vi "getAllRefs.vi"(8 "error in (no error)":errorcluster, 10 "Language":u8, 11 "Change Language":bool) -> (0 "error out":errorcluster, 3 "Control references [ ]":T1(array[cluster]))   [LabVIEW 2013, in "main.lvlib"]
uses:
  main.lvlib
  <userlib>/_OpenG.lib/file/file.llb/File Exists - Scalar__ogtk.vi
  <vilib>/Utility/file.llb/Read From Spreadsheet File (string).vi
  <vilib>/Utility/file.llb/Write To Spreadsheet File (string).vi
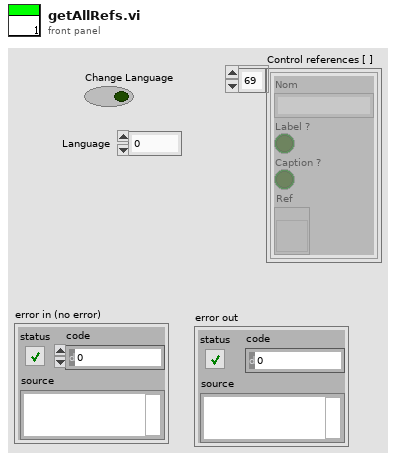
[diagram p1: front panel]
types:
  T1 = cluster{"Nom":string, "Label ?":bool, "Caption ?":bool, "Ref":refnum<vi>}[]
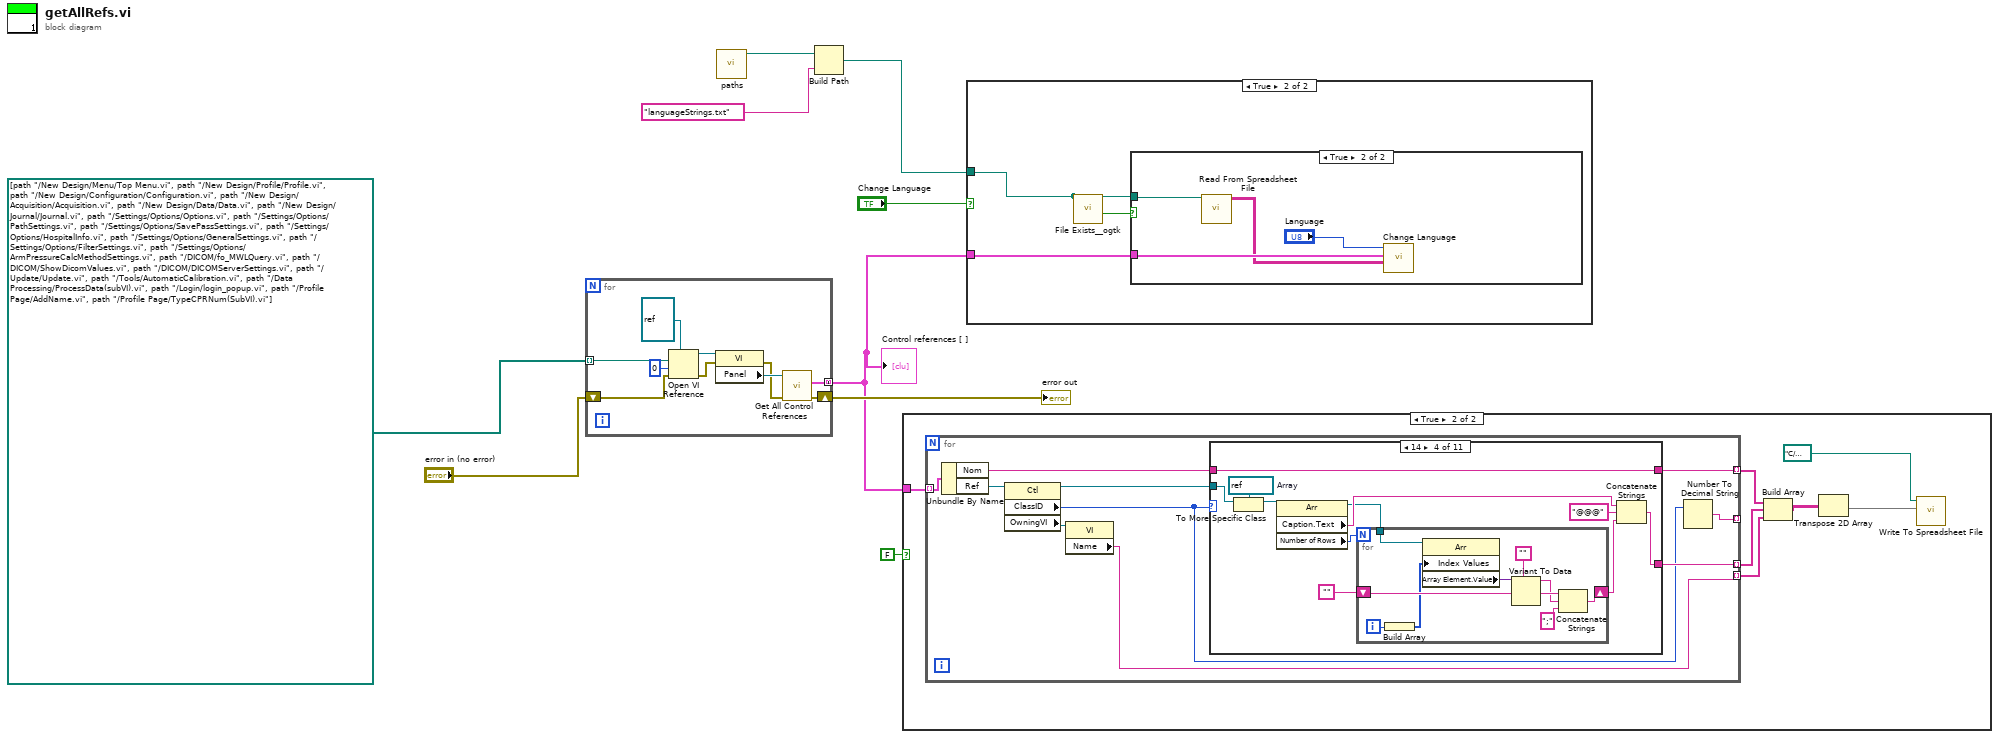
[diagram p0: block diagram]
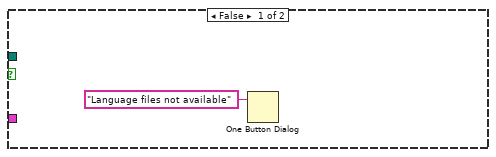
[diagram p3: hidden frame]
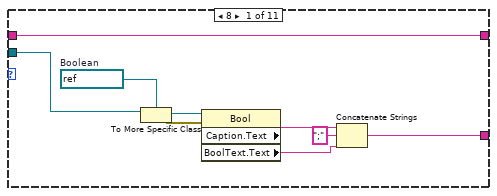
[diagram p5: hidden frame]
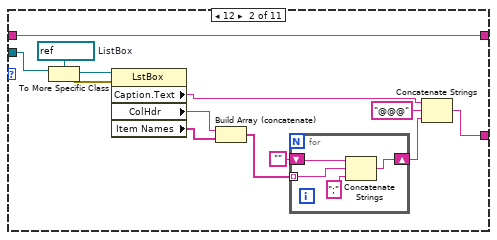
[diagram p6: hidden frame]
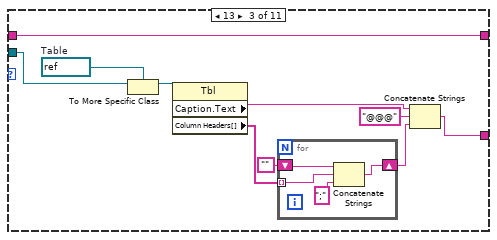
[diagram p7: hidden frame]
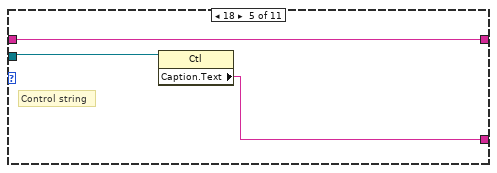
[diagram p8: hidden frame]
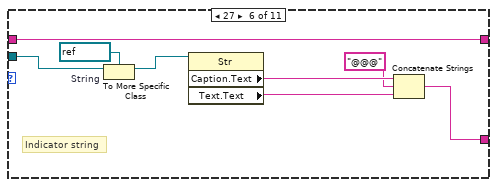
[diagram p9: hidden frame]
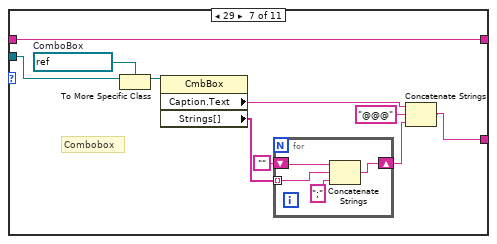
[diagram p10: hidden frame]
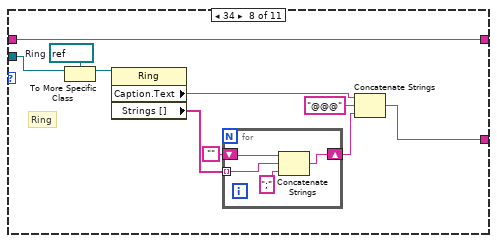
[diagram p11: hidden frame]
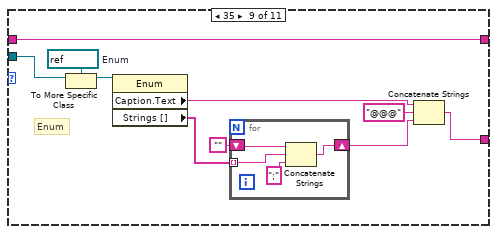
[diagram p12: hidden frame]
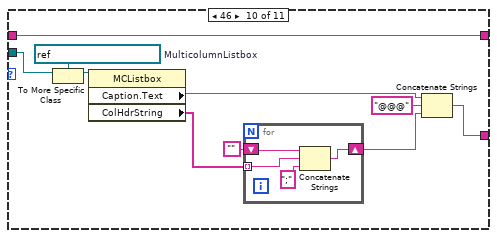
[diagram p13: hidden frame]
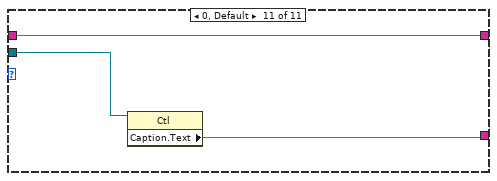
[diagram p14: hidden frame]
diagram:
  n1 = for {
    tunnel: [w14] -> w5 mode=concatenating
    tunnel: path[] [path "../New Design/Menu/Top Menu.vi", path "../New Design/Profile/Profile.vi", path "../New Design/Configuration/Configuration.vi", path "../New Design/Acquisition/Acquisition.vi", path "../New Design/Data/Data.vi", path "../New Design/Journal/Journal.vi", path "../Settings/Options/Options.vi", path "../Settings/Options/PathSettings.vi", path "../Settings/Options/SavePassSettings.vi", path "../Settings/Options/HospitalInfo.vi", path "../Settings/Options/GeneralSettings.vi", path "../Settings/Options/FilterSettings.vi", path "../Settings/Options/ArmPressureCalcMethodSettings.vi", path "../DICOM/fo_MWLQuery.vi", path "../DICOM/ShowDicomValues.vi", path "../DICOM/DICOMServerSettings.vi", path "../Update/Update.vi", path "../Tools/AutomaticCalibration.vi", path "../Data Processing/ProcessData(subVI).vi", path "../Login/login_popup.vi", path "../Profile Page/AddName.vi", path "../Profile Page/TypeCPRNum(SubVI).vi"] -> [w15] mode=indexing
    shift-right: [w10] -> w7
    shift-left: "error in (no error)" -> [w13]
    n2 = Open VI Reference(type specifier VI Refnum (for type only)=refnum<vi> refnum, vi path=w15, options=0, error in (no error)=w13) -> (vi reference=w17:refnum<vi>, error out=w12:errorcluster)  [unwired: 2 in]
    n3 = property class="VI"(reference=w17, error in=w12) -> (error out=w11:errorcluster, "Panel"=w16:refnum<vi>)  [unwired: 1 out]
    n4 = call "Get All Control References.vi"("error in (no error)"=w11, "Panel refnum"=w16) -> ("error out"=w10:errorcluster, "Control references [ ]"=w14:T1)  [unwired: 5 in, 1 out]
  }
  "error out" <- w7
  "Control references [ ]" <- w5
  n5 = call "paths.vi"() -> ("PubAppData"=w3:path)  [unwired: 8 in, 3 out]
  n6 = Build Path(base path=w3, name or relative path="languageStrings.txt") -> (appended path=w1:path)
  n7 = case shown="True" FALSE {
    tunnel: w5 -> [_ w26]
    frame False {
    }
    frame True {
      n8 = for {
        tunnel: w26 -> [w36] mode=indexing
        tunnel: [w31] -> w24 mode=indexing
        tunnel: [w33] -> w23 mode=indexing
        tunnel: [w29] -> _ mode=indexing
        tunnel: [w27] -> w20 mode=indexing
        n9 = Unbundle By Name(w36) -> ("Nom"=w32:string, "Ref"=w35:refnum<vi>)
        n10 = property class="Ctl"(reference=w35) -> (reference out=w34:refnum<vi>, "ClassID"=w30:u32, "OwningVI"=w28:refnum<vi>)  [unwired: 1 in, 1 out]
        n11 = property class="VI"(reference=w28) -> ("Name"=w27:string)  [unwired: 1 in, 2 out]
        n12 = case shown="14" w30 {
          tunnel: w34 -> [w45 w55 w71 w86 w98 w105 w115 w126 w143 w154 w166]
          tunnel: [w38 w49 w63 w79 w97 w102 w110 w125 w139 w152 w165] -> w33
          tunnel: w32 -> [w37 w54 w70 w85 w99 w107 w114 w124 w142 w155 w164]
          tunnel: [w37 w54 w70 w85 w99 w107 w114 w124 w142 w155 w164] -> w31
          frame 8 {
            w44 = refnum<vi> refnum  # Boolean
            n13 = To More Specific Class(target class=w44, reference=w45) -> (specific class reference=w43:refnum<vi>, error out=w42:errorcluster)  [unwired: 1 in]
            n14 = property class="Bool"(reference=w43, error in=w42) -> ("Caption.Text"=w41:string, "BoolText.Text"=w39:string)  [unwired: 2 out]
            n15 = Concatenate Strings(w41, ";" ("string"), w39) -> (w38:string)
          }
          frame 12 {
            w58 = refnum<vi> refnum  # ListBox
            n16 = To More Specific Class(target class=w58, reference=w55) -> (specific class reference=w57:refnum<vi>, error out=w56:errorcluster)  [unwired: 1 in]
            n17 = property class="LstBox"(reference=w57, error in=w56) -> ("Caption.Text"=w50:string, "ColHdr"=w48:string, "Item Names"=w47:string[])  [unwired: 2 out]
            n18 = Build Array (concatenate)(w48, w47) -> (w46:string[])
            n19 = for {
              shift-right: [w61] -> w52
              shift-left: "" -> [w62]
              tunnel: w46 -> [w60] mode=indexing
              n20 = Concatenate Strings(w62, w60, ";" ("string")) -> (w61:string)
            }
            n21 = Concatenate Strings(w50, "@@@" ("string"), w52) -> (w49:string)
          }
          frame 13 {
            w72 = refnum<vi> refnum  # Table
            n22 = To More Specific Class(target class=w72, reference=w71) -> (specific class reference=w69:refnum<vi>)  [unwired: 1 in, 1 out]
            n23 = property class="Tbl"(reference=w69) -> ("Caption.Text"=w65:string, "Column Headers[]"=w64:string[])  [unwired: 1 in, 2 out]
            n24 = for {
              shift-right: [w75] -> w67
              shift-left: "" -> [w76]
              tunnel: w64 -> [w74] mode=indexing
              n25 = Concatenate Strings(w76, w74, ";" ("string")) -> (w75:string)
            }
            n26 = Concatenate Strings(w65, "@@@" ("string"), w67) -> (w63:string)
          }
          frame 14 {
            w87 = refnum<vi> refnum  # Array
            n27 = To More Specific Class(target class=w87, reference=w86) -> (specific class reference=w84:refnum<vi>)  [unwired: 1 in, 1 out]
            n28 = property class="Arr"(reference=w84) -> (reference out=w77:refnum<vi>, "Caption.Text"=w80:string, "Number of Rows"=w78:u32)  [unwired: 1 in, 1 out]
            n29 = for {
              N: w78 -> [_]
              shift-right: [w95] -> w82
              shift-left: "" -> [w96]
              tunnel: w77 -> [w93]
              i -> [w92]
              n30 = Build Array(w92) -> (w91:i32[])
              n31 = property class="Arr"(reference=w93, "Index Values"=w91) -> ("Array Element.Value"=w90:variant)  [unwired: 1 in, 2 out]
              n32 = Variant To Data(type="", Variant=w90) -> (data=w88:string)  [unwired: 1 in, 1 out]
              n33 = Concatenate Strings(w96, w88, ";" ("string")) -> (w95:string)
            }
            n34 = Concatenate Strings(w80, "@@@" ("string"), w82) -> (w79:string)
          }
          frame 18 {
            # "Control string"
            n35 = property class="Ctl"(reference=w98) -> ("Caption.Text"=w97:string)  [unwired: 1 in, 2 out]
          }
          frame 27 {
            w106 = refnum<vi> refnum  # String
            # "Indicator string"
            n36 = To More Specific Class(target class=w106, reference=w105) -> (specific class reference=w104:refnum<vi>)  [unwired: 1 in, 1 out]
            n37 = property class="Str"(reference=w104) -> ("Caption.Text"=w103:string, "Text.Text"=w101:string)  [unwired: 1 in, 2 out]
            n38 = Concatenate Strings(w103, "@@@" ("string"), w101) -> (w102:string)
          }
          frame 29 {
            w117 = refnum<vi> refnum  # ComboBox
            # "Combobox"
            n39 = To More Specific Class(target class=w117, reference=w115) -> (specific class reference=w116:refnum<vi>)  [unwired: 1 in, 1 out]
            n40 = property class="CmbBox"(reference=w116) -> ("Caption.Text"=w109:string, "Strings[]"=w108:string[])  [unwired: 1 in, 2 out]
            n41 = for {
              shift-right: [w120] -> w112
              shift-left: "" -> [w121]
              tunnel: w108 -> [w119] mode=indexing
              n42 = Concatenate Strings(w121, w119, ";" ("string")) -> (w120:string)
            }
            n43 = Concatenate Strings(w109, "@@@" ("string"), w112) -> (w110:string)
          }
          frame 34 {
            w131 = refnum<vi> refnum  # Ring
            # "Ring"
            n44 = To More Specific Class(target class=w131, reference=w126) -> (specific class reference=w130:refnum<vi>)  [unwired: 1 in, 1 out]
            n45 = property class="Ring"(reference=w130) -> ("Caption.Text"=w123:string, "Strings []"=w129:string[])  [unwired: 1 in, 2 out]
            n46 = for {
              shift-right: [w134] -> w127
              shift-left: "" -> [w135]
              tunnel: w129 -> [w133] mode=indexing
              n47 = Concatenate Strings(w135, w133, ";" ("string")) -> (w134:string)
            }
            n48 = Concatenate Strings(w123, "@@@" ("string"), w127) -> (w125:string)
          }
          frame 35 {
            w145 = refnum<vi> refnum  # Enum
            # "Enum"
            n49 = To More Specific Class(target class=w145, reference=w143) -> (specific class reference=w144:refnum<vi>)  [unwired: 1 in, 1 out]
            n50 = property class="Enum"(reference=w144) -> ("Caption.Text"=w140:string, "Strings []"=w137:string[])  [unwired: 1 in, 2 out]
            n51 = for {
              shift-right: [w148] -> w136
              shift-left: "" -> [w149]
              tunnel: w137 -> [w147] mode=indexing
              n52 = Concatenate Strings(w149, w147, ";" ("string")) -> (w148:string)
            }
            n53 = Concatenate Strings(w140, "@@@" ("string"), w136) -> (w139:string)
          }
          frame 46 {
            w159 = refnum<vi> refnum  # MulticolumnListbox
            n54 = To More Specific Class(target class=w159, reference=w154) -> (specific class reference=w158:refnum<vi>)  [unwired: 1 in, 1 out]
            n55 = property class="MCListbox"(reference=w158) -> ("Caption.Text"=w156:string, "ColHdrString"=w151:string[])  [unwired: 1 in, 2 out]
            n56 = for {
              shift-right: [w162] -> w153
              shift-left: "" -> [w163]
              tunnel: w151 -> [w161] mode=indexing
              n57 = Concatenate Strings(w163, w161, ";" ("string")) -> (w162:string)
            }
            n58 = Concatenate Strings(w156, "@@@" ("string"), w153) -> (w152:string)
          }
          frame 0, Default {
            n59 = property class="Ctl"(reference=w166) -> ("Caption.Text"=w165:string)  [unwired: 1 in, 2 out]
          }
        }
        n60 = Number To Decimal String(number=w30) -> (decimal integer string=w29:string)  [unwired: 1 in]
      }
      n61 = Build Array(w24, w23, w20) -> (w25:string[][])
      n62 = Transpose 2D Array(2D array=w25) -> (transposed array=w21:string[][])
      n63 = call-poly <vilib>:"Write To Spreadsheet File.vi"("2D data"=w21, "file path (dialog if empty)"=path "C:/Users/simon/SkyDrive/LabView/2013/DM2020/Language/allRefs.txt") -> ()  [unwired: 6 in, 1 out]
    }
  }
  n64 = case shown="True" "Change Language" {
    tunnel: w5 -> [_ w169]
    tunnel: w1 -> [_ w167]
    frame False {
    }
    frame True {
      n65 = call-poly <userlib>:"File Exists__ogtk.vi"("file path"=w167) -> ("exists"=w168:bool)  [unwired: 6 in, 1 out]
      n66 = case shown="True" w168 {
        tunnel: w169 -> [_ w174]
        tunnel: w167 -> [_ w171]
        frame False {
          n67 = One Button Dialog(message="Language files not available") -> ()  [unwired: 1 in, 1 out]
        }
        frame True {
          n68 = call-poly <vilib>:"Read From Spreadsheet File.vi"("file path (dialog if empty)"=w171) -> ("all rows"=w173:string[][])  [unwired: 6 in, 4 out]
          n69 = call "Change Language.vi"("Array IN"=w173, "References Pane"=w174, "Langues/Languages"="Language") -> ()  [unwired: 9 in]
        }
      }
    }
  }
